vi "Generador_Senal_conv.vi"(8 "Vertical Fill Slide":dbl(slide) scale=-4.0..4.0, 9 "df":dbl, 10 "to":dbl, 11 "tf":dbl) -> (0 "Tiempo 2":dbl[](array[numeric]), 1 "X2":dbl[](array[numeric]), 2 "X1":dbl[](array[numeric]), 3 "Tiempo":dbl[](array[numeric]))   [LabVIEW 2017]
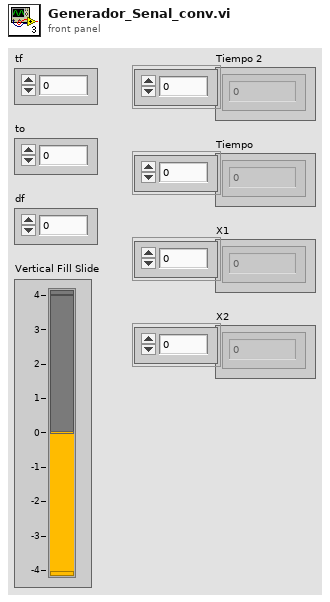
[diagram p1: front panel]
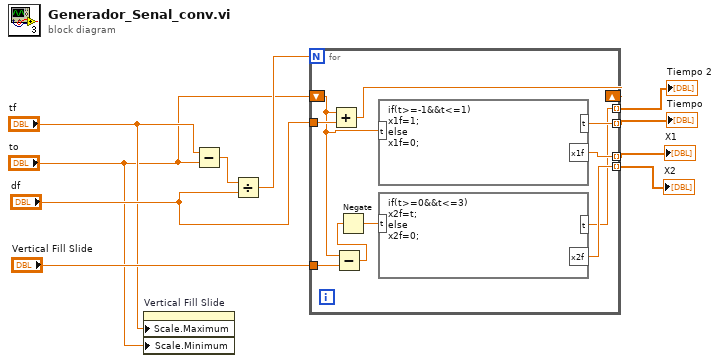
[diagram p0: block diagram]
diagram:
  n1 = property on="Vertical Fill Slide" class="Slide (strict)"("Scale.Maximum"="tf", "Scale.Minimum"="to") -> ()  [unwired: 2 in, 2 out]
  n2 = Subtract(x="tf", y="to") -> (x-y=w3:dbl)
  n3 = Divide(x=w3, y="df") -> (x/y=w4:dbl)
  n4 = for {
    N: w4 -> [_]
    shift-right: [w20] -> _
    shift-left: "to" -> [w14]
    tunnel: "df" -> [w19]
    tunnel: [w18] -> w7 mode=indexing
    tunnel: [w17] -> w9 mode=indexing
    tunnel: [w16] -> w8 mode=indexing
    tunnel: "Vertical Fill Slide" -> [w15]
    tunnel: [w11] -> w10 mode=indexing
    n5 = Add(x=w14, y=w19) -> (x+y=w20:dbl)
    n6 = Subtract(x=w14, y=w15) -> (x-y=w13:dbl)
    n7 = Negate(x=w13) -> (-x=w12:dbl)
    n8 = formula code="if(t>=-1&&t<=1)\nx1f=1;\nelse\nx1f=0;"("t"=w14) -> ("x1f"=w18:dbl, "t"=w17:dbl)
    n9 = formula code="if(t>=0&&t<=3)\nx2f=t;\nelse\nx2f=0;"("t"=w12) -> ("x2f"=w16:dbl, "t"=w11:dbl)
  }
  "Tiempo" <- w9
  "X1" <- w7
  "X2" <- w8
  "Tiempo 2" <- w10
